vi "写入命令.vi"(8 "error in (no error)":errorcluster caption="错误输入（无错误）", 10 "字符串":string, 11 "消息类 输入":refnum<class "消息类.lvclass">) -> (0 "error out":errorcluster caption="错误输出", 3 "消息类 输出":refnum<class "消息类.lvclass">)   [LabVIEW 2016, in "消息类.lvclass"]
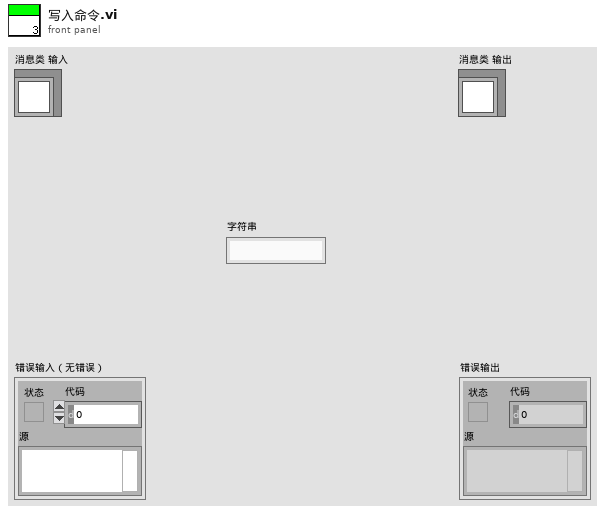
[diagram p1: front panel]
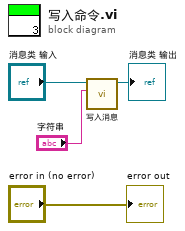
[diagram p0: block diagram]
diagram:
  n1 = call-dynamic "写入消息.vi"("消息"="字符串", "消息类输入"="消息类 输入") -> ("消息类输出"=→"消息类 输出":refnum<class "消息类.lvclass">)  [unwired: 8 in, 1 out]
  "error out" <- "error in (no error)"
